vi "Radian to Degree.vi"(11 "Radians":dbl) -> (3 "Degrees":dbl)   [LabVIEW 2014]
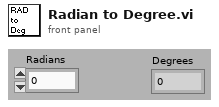
[diagram p1: front panel]
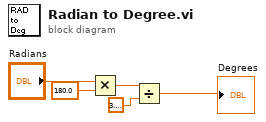
[diagram p0: block diagram]
diagram:
  n1 = Multiply(x="Radians", y=180.0) -> (x*y=w3:dbl)
  n2 = Divide(x=w3, y=3.141592653589793) -> (x/y=→"Degrees":dbl)
